vi "SP Convert Limits Points to MHz.vi"(4 "Units":T7, 5 "Limits In":T1[](array[typedef]) {"Parameter"."Stimulus Port" min=1 step=1; "Parameter"."Response Port" min=1 step=1}) -> (1 "Limits Out":T1[](array[typedef]) {"Parameter"."Stimulus Port" min=1 step=1; "Parameter"."Response Port" min=1 step=1})   [LabVIEW 2011]
uses:
  TypeDefs/SP Limit.ctl
  TypeDefs/SP Parameter.ctl
  TypeDefs/SP Format.ctl
  TypeDefs/SP Limit Type.ctl
  TypeDefs/SP Limit Point.ctl
  Test Referential Limit.ctl
  TypeDefs/SP Frequency Units.ctl
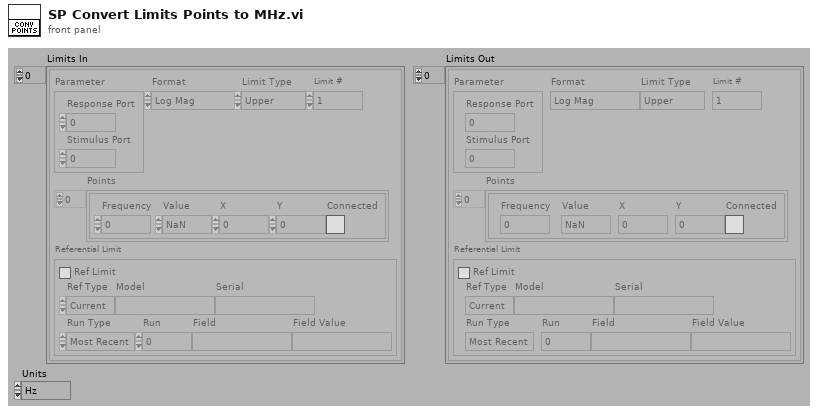
[diagram p1: front panel]
types:
  T1 = typedef "SP Limit.ctl" = cluster{"Parameter":T2, "Format":T3, "Limit Type":T4, "Points":T5[], "Referential Limit":T6, "Limit #":i8}
  T2 = typedef "SP Parameter.ctl" = cluster{"Stimulus Port":i8, "Response Port":i8}
  T3 = typedef "SP Format.ctl" = enum16{"Log Mag", "Lin Mag", "SWR", "Phase", "Expanded Phase", "Delay", "Insertion Loss", "Isolation", "Return Loss"}
  T4 = typedef "SP Limit Type.ctl" = enum16{"Upper", "Lower", "Delta", "Filter", "Referential"}
  T5 = typedef "SP Limit Point.ctl" = cluster{"Frequency":dbl, "Value":dbl, "X":dbl, "Y":dbl, "Connected":bool}
  T6 = typedef "Test Referential Limit.ctl" = cluster{"Ref Limit":bool, "Ref Type":enum16{"Current", "Specify"}, "Model":string, "Serial":string, "Run Type":enum16{"Most Recent", "Run #", "Match Field"}, "Run":i32, "Field":string, "Field Value":string}
  T7 = typedef "SP Frequency Units.ctl" = enum16{"Hz", "kHz", "MHz", "GHz", "Points"}
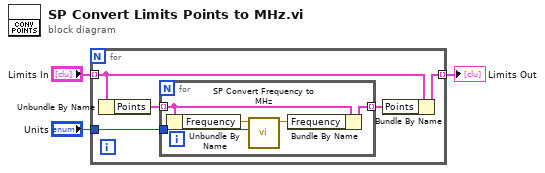
[diagram p0: block diagram]
diagram:
  n1 = for {
    tunnel: "Limits In" -> [w7] mode=indexing
    tunnel: [w5] -> w3 mode=indexing
    tunnel: "Units" -> [w4]
    n2 = Unbundle By Name(w7) -> ("Points"=w8:T5[])
    n3 = for {
      tunnel: w8 -> [w12] mode=indexing
      tunnel: [w10] -> w6 mode=indexing
      tunnel: w4 -> [w9]
      n4 = Unbundle By Name(w12) -> ("Frequency"=w13:dbl)
      n5 = call "SP Convert Frequency to MHz.vi"("Units"=w9, "Frequency"=w13) -> ("Converted Frequency"=w11:dbl)  [unwired: 1 in, 8 out]
      n6 = Bundle By Name(cluster=w12, "Frequency"=w11) -> (w10:T5)
    }
    n7 = Bundle By Name(cluster=w7, "Points"=w6) -> (w5:T1)
  }
  "Limits Out" <- w3
